vi "01_Main.vi"() -> ()   [LabVIEW 2020]
doc: "This is the Main VI that I use when testing console communication testing.\n\nThis simulates an LPCA by responding to the commands sent by the console."
uses:
  <vilib>/DAQmx/write.llb/DAQmx Write (Digital Bool 1Line 1Point).vi
  <vilib>/DAQmx/read.llb/DAQmx Read (Digital Bool 1Line 1Point).vi
  <vilib>/Instr/_visa.llb/VISA Configure Serial Port (Serial Instr).vi
  <vilib>/DAQmx/miscellaneous.llb/DAQmx Fill In Error Info.vi
panel:
  out "MSTOP STOP":bool
  in  "MSTOP REL":bool
  in  "MSTOP PWR":bool=TRUE
  out "Waveform Chart":u32(graph)
  out "Err32?":bool
  in  "stop":bool
  in  "VISA resource name":refnum<visa-resource-name>
  # "IMPORTANT:\nMake sure to se the COM port in the VISA resource name before starting this VI."
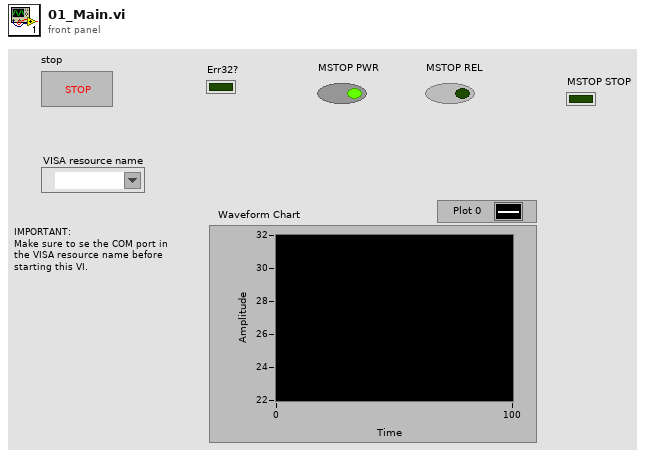
[diagram p1: front panel]
types:
  T1 = enum16{"Init", "Read", "Obs On", "Obs Off", "MStop On", "MStop Off"}
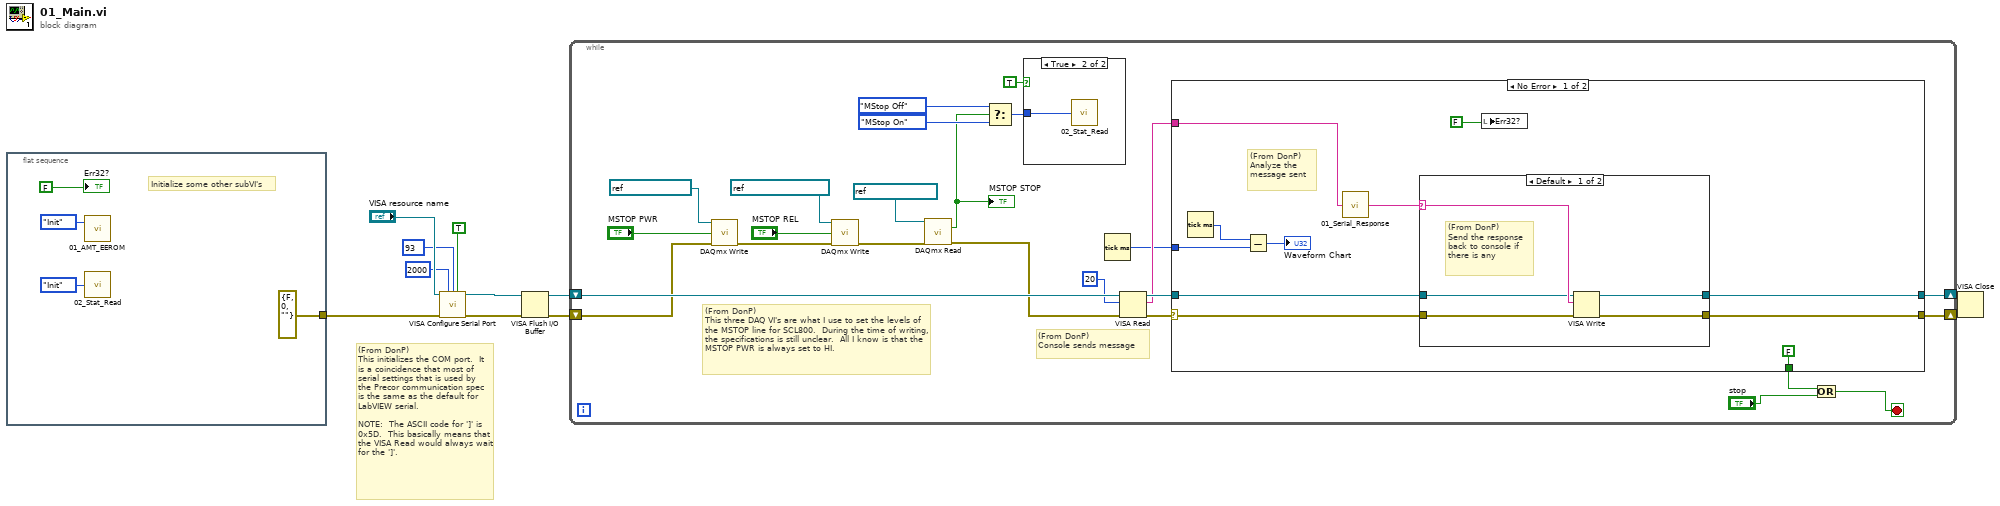
[diagram p0: block diagram]
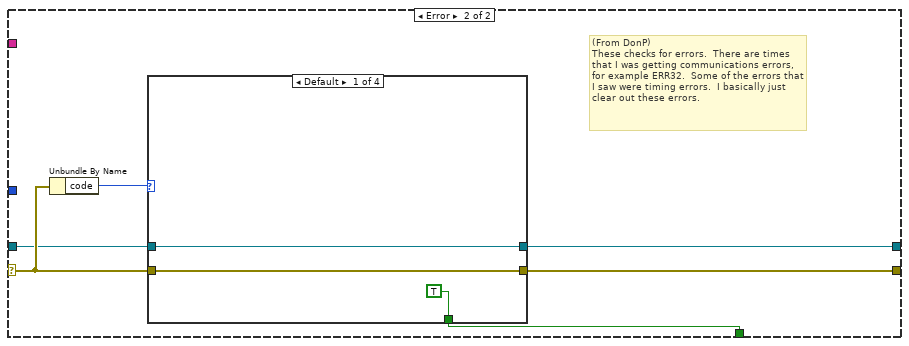
[diagram p4: hidden frame]
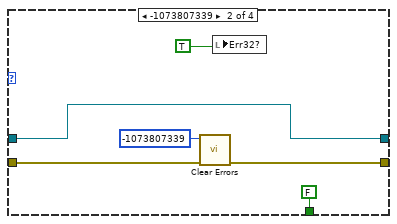
[diagram p5: hidden frame]
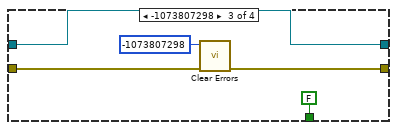
[diagram p6: hidden frame]
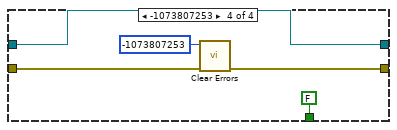
[diagram p7: hidden frame]
diagram:
  # "(From DonP)\nThis initializes the COM port.  It is a coincidence that most of serial settings that is used by the Precor communication spec is the same as the default for LabVIEW serial.\n\nNOTE:  The ASCII code for ']' is 0x5D.  This basically means that the VISA Read would always wait for the ']'."
  n1 = flat-sequence {
    tunnel: [errorcluster {"status"=FALSE, "code"=0, "source"=""} ("error constant")] -> w1
    frame #0 {
      # "Initialize some other subVI's"
      n2 = call "01_AMT_EEROM.vi"("Command"=enum16{"Init", "EERD", "EEWR"}."Init") -> ()  [unwired: 2 in, 1 out]
      n3 = call "02_Stat_Read.vi"("Command"=T1."Init") -> ()  [unwired: 1 out]
      "Err32?" <- FALSE ("Err32?")
    }
  }
  n4 = call-poly "VISA Configure Serial Port"("VISA resource name"="VISA resource name", "timeout (10sec)"=u32 2000, "termination char\n(0xA = '\\n' = LF)"=u8 93 ("termination char\n(0xA = '\\n' = LF)"), "Enable Termination\nChar (T)"=TRUE ("Enable Termination\nChar (T)"), "error in (no error)"=w1) -> ("VISA resource name out"=w5:refnum<visa-resource-name>, "error out"=w4:errorcluster)  [unwired: 9 in]
  n5 = VISA Flush I/O Buffer(VISA resource name=w5, error in (no error)=w4) -> (VISA resource name out=w2:refnum<visa-resource-name>, error out=w3:errorcluster)  [unwired: 1 in]
  n6 = while {
    shift-right: [w35] -> w9
    shift-left: w2 -> [w40]
    shift-right: [w36] -> w8
    shift-left: w3 -> [w28]
    stop <- w32 stop-if-true
    # "(From DonP)\nConsole sends message"
    # "(From DonP)\nThis three DAQ VI's are what I use to set the levels of the MSTOP line for SCL800.  During the time of writing, the specifications is still unclear.  All I know is that the MSTOP PWR is always set to HI."
    n7 = call-poly <vilib>:"DAQmx Write.vi"("task/channels in"=refnum<k21> "MSTOP_PWR", "data"="MSTOP PWR", "error in"=w28) -> ("error out"=w26:errorcluster)  [unwired: 10 in, 2 out]
    n8 = call-poly <vilib>:"DAQmx Write.vi"("task/channels in"=refnum<k21> "MSTOP_RELEASE", "data"="MSTOP REL", "error in"=w26) -> ("error out"=w23:errorcluster)  [unwired: 10 in, 2 out]
    n9 = call-poly <vilib>:"DAQmx Read.vi"("task/channels in"=refnum<k21> "MSTOP_STOP", "error in"=w23) -> ("data"=w17:bool, "error out"=w21:errorcluster)  [unwired: 11 in, 1 out]
    "MSTOP STOP" <- w17
    n10 = Select(t=T1."MStop Off" ("Command"), s=w17, f=T1."MStop On" ("Command")) -> (s? t:f=w20:T1)
    n11 = case shown="True" TRUE {
      tunnel: w20 -> [_ w41]
      frame False {
      }
      frame True {
        n12 = call "02_Stat_Read.vi"("Command"=w41) -> ()  [unwired: 1 out]
      }
    }
    n13 = Tick Count (ms)() -> (millisecond timer value=w31:u32)
    n14 = VISA Read(VISA resource name=w40, byte count=u32 20, error in (no error)=w21) -> (VISA resource name out=w39:refnum<visa-resource-name>, read buffer=w37:string, error out=w38:errorcluster)  [unwired: 1 out]
    n15 = case shown="No Error" w38 {
      selector: w38 -> [w48 w64]
      tunnel: w39 -> [w49 w63]
      tunnel: w37 -> [w51 _]
      tunnel: [w46 w62] -> w36
      tunnel: [w47 w61] -> w35
      tunnel: [FALSE w60] -> w33
      tunnel: w31 -> [w43 _]
      frame No Error {
        # "(From DonP)\nAnalyze the message sent"
        n16 = Tick Count (ms)() -> (millisecond timer value=w44:u32)
        n17 = Subtract(x=w44, y=w43) -> (x-y=→"Waveform Chart":u32)
        n18 = call "01_Serial_Response.vi"("Read"=w51) -> ("Response"=w50:string)  [unwired: 4 in]
        n19 = case shown="Default" w50 {
          selector: w50 -> [w57 _]
          tunnel: w49 -> [w56 w59]
          tunnel: w48 -> [w55 w58]
          tunnel: [w54 w59] -> w47
          tunnel: [w53 w58] -> w46
          frame Default {
            # "(From DonP)\nSend the response back to console if there is any"
            n20 = VISA Write(VISA resource name=w56, write buffer=w57, error in (no error)=w55) -> (VISA resource name out=w54:refnum<visa-resource-name>, error out=w53:errorcluster)  [unwired: 1 out]
          }
          frame "" {
          }
        }
        n21 = local write "Err32?"(FALSE ("Err32?")) -> ()
      }
      frame Error {
        # "(From DonP)\nThese checks for errors.  There are times that I was getting communications errors, for example ERR32.  Some of the errors that I saw were timing errors.  I basically just clear out these errors."
        n22 = Unbundle By Name(w64) -> ("code"=w65:i32)
        n23 = case shown="Default" w65 {
          tunnel: w64 -> [w68 w73 w78 w83]
          tunnel: w63 -> [w67 w71 w76 w81]
          tunnel: [w68 w70 w75 w80] -> w62
          tunnel: [w67 w71 w76 w81] -> w61
          tunnel: [TRUE FALSE FALSE FALSE] -> w60
          frame Default {
          }
          frame -1073807339 {
            n24 = call <vilib>:"Clear Errors.vi"("error in (no error)"=w73, "specific error code to clear (0: all)"=-1073807339) -> ("error out"=w70:errorcluster)  [unwired: 4 in, 1 out]
            n25 = local write "Err32?"(TRUE ("Err32?")) -> ()
          }
          frame -1073807298 {
            n26 = call <vilib>:"Clear Errors.vi"("error in (no error)"=w78, "specific error code to clear (0: all)"=-1073807298) -> ("error out"=w75:errorcluster)  [unwired: 4 in, 1 out]
          }
          frame -1073807253 {
            n27 = call <vilib>:"Clear Errors.vi"("error in (no error)"=w83, "specific error code to clear (0: all)"=-1073807253) -> ("error out"=w80:errorcluster)  [unwired: 4 in, 1 out]
          }
        }
      }
    }
    n28 = Or(x=w33, y="stop") -> (x .or. y?=w32:bool)
  }
  n29 = VISA Close(VISA resource name=w9, error in (no error)=w8) -> ()  [unwired: 1 out]
